vi "WPI_RelayCache.vi"(7 "Operation":T3, 8 "error in (no error)":errorcluster, 9 "RelayDirection":T1, 11 "RelayChannelIn":T2) -> (0 "error out":errorcluster, 2 "Allocated":bool, 3 "RelayChannelOut":T2)   [LabVIEW 2017]
doc: "This software is licensed. Open the labview\\readme\\WPI Robotics Library Open Source License.txt file for more information."
uses:
  <vilib>/Rock Robotics/WPI/Relay/WPI_RelayCacheOp.ctl
  <vilib>/Rock Robotics/SystemInterfaces/DIO/FPGA_DIORelayChannel.ctl
  <vilib>/Rock Robotics/WPI/Relay/WPI_RelayDirection.ctl
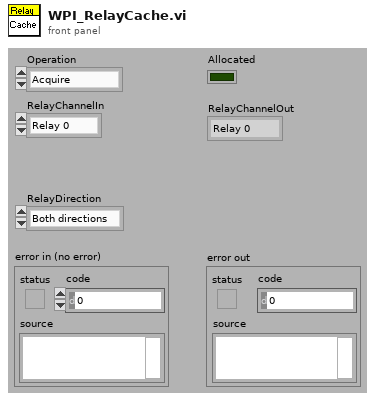
[diagram p1: front panel]
types:
  T1 = typedef "WPI_RelayDirection.ctl" = enum16{"Both directions", "Forward only", "Reverse only"}
  T2 = typedef "FPGA_DIORelayChannel.ctl" = enum8{"Relay 0", "Relay 1", "Relay 2", "Relay 3", "Invalid"}
  T3 = typedef "WPI_RelayCacheOp.ctl" = enum16{"Acquire", "Release", "Status"}
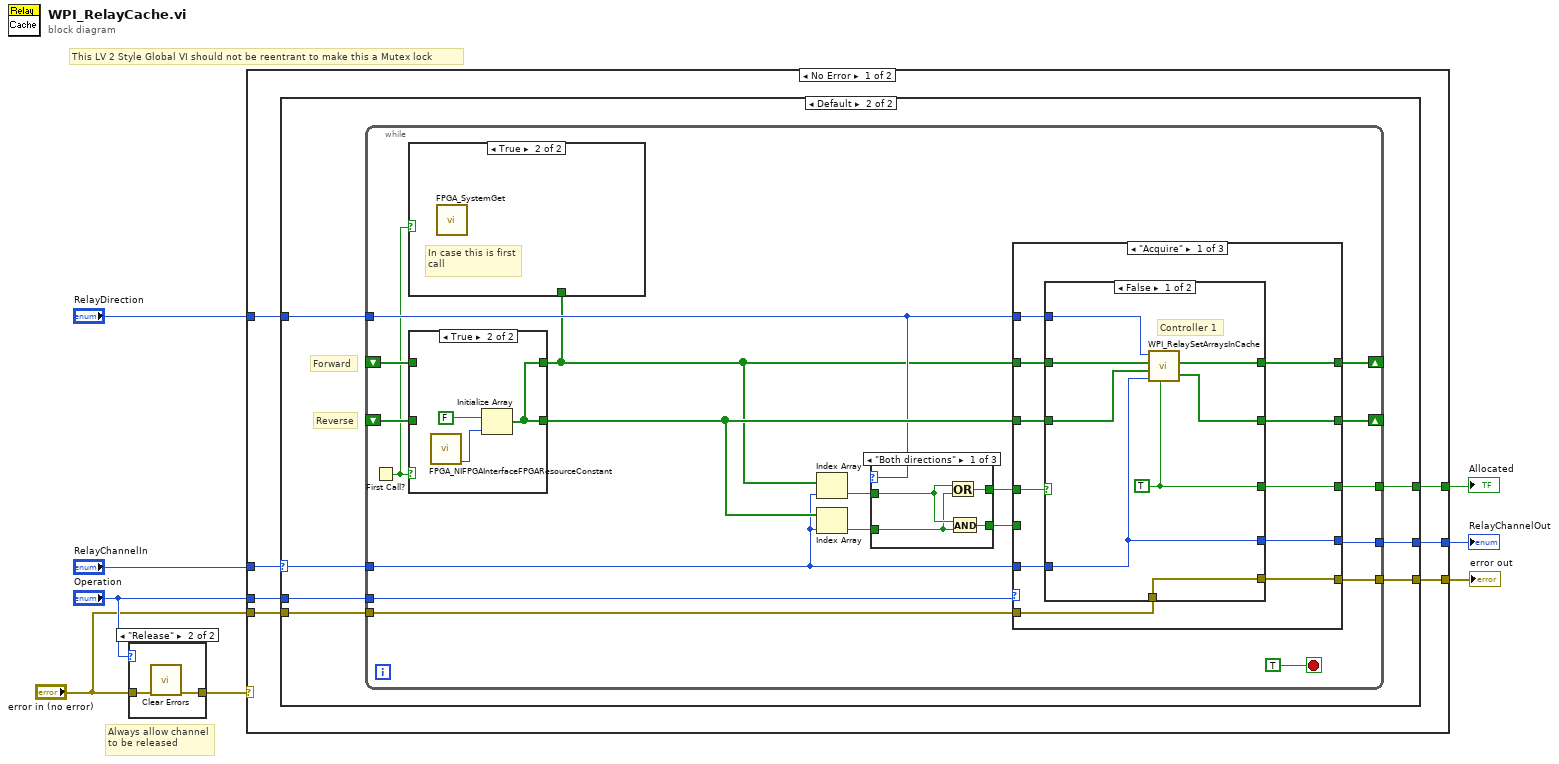
[diagram p0: block diagram]
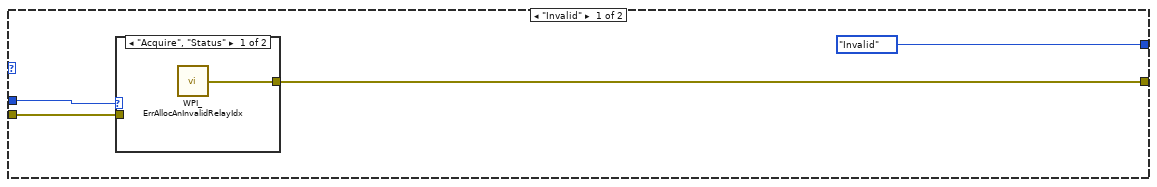
[diagram p2: hidden frame]
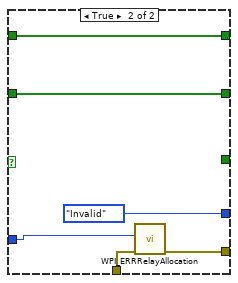
[diagram p6: hidden frame]
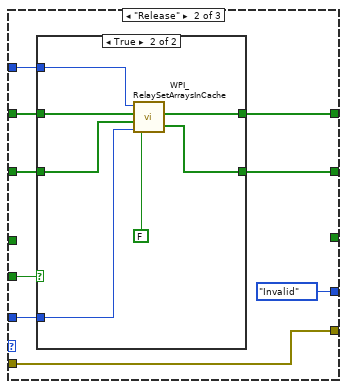
[diagram p7: hidden frame]
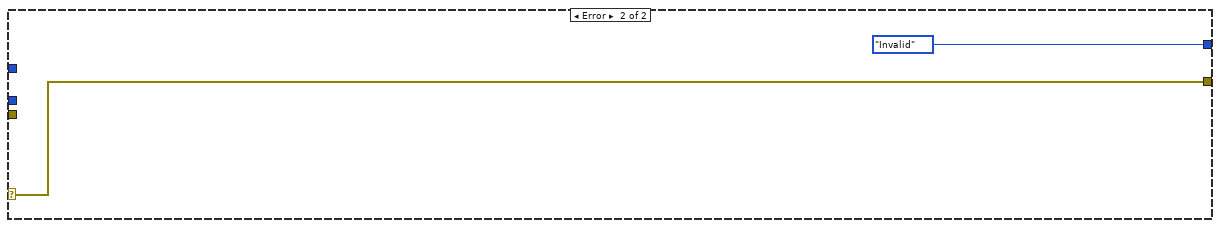
[diagram p12: hidden frame]
diagram:
  # "This LV 2 Style Global VI should not be reentrant to make this a Mutex lock"
  # "Always allow channel to be released"
  n1 = case shown="\"Release\"" "Operation" {
    tunnel: "error in (no error)" -> [w9 w11]
    tunnel: [w9 w10] -> w8
    frame "Acquire", Default {
    }
    frame "Release" {
      n2 = call <vilib>:"Clear Errors.vi"("error in (no error)"=w11) -> ("error out"=w10:errorcluster)  [unwired: 1 in, 5 out]
    }
  }
  n3 = case shown="No Error" w8 {
    selector: w8 -> [_ w110]
    tunnel: "Operation" -> [w18 _]
    tunnel: "RelayChannelIn" -> [w17 _]
    tunnel: [w16 w110] -> w1
    tunnel: [w15 _] -> w5
    tunnel: [w14 FPGA_DIORelayChannel."Invalid" ("RelayChannelOut")] -> w4
    tunnel: "RelayDirection" -> [w13 _]
    tunnel: "error in (no error)" -> [w12 _]
    frame No Error {
      n4 = case shown="Default" w17 {
        selector: w17 -> [_ w26]
        tunnel: w18 -> [w21 w30]
        tunnel: [w20 w29] -> w16
        tunnel: [_ w28] -> w15
        tunnel: [FPGA_DIORelayChannel."Invalid" ("RelayChannelOut") w27] -> w14
        tunnel: w13 -> [_ w25]
        tunnel: w12 -> [w19 w24]
        frame "Invalid" {
          n5 = case shown="\"Acquire\", \"Status\"" w21 {
            tunnel: [w23 _] -> w20
            tunnel: w19 -> [_ _]
            frame "Acquire", "Status" {
              n6 = call <vilib>:"WPI_ErrAllocAnInvalidRelayIdx.vi"() -> ("error out"=w23:errorcluster)
            }
            frame "Release" {
            }
          }
        }
        frame Default {
          # "Forward"
          # "Reverse"
          n7 = while {
            shift-right: [w47] -> _
            shift-left: _ -> [w49]
            tunnel: w30 -> [w48]
            tunnel: w26 -> [w38]
            tunnel: [w46] -> w29
            tunnel: [w45] -> w28
            tunnel: [w42] -> w27
            shift-right: [w40] -> _
            shift-left: _ -> [w41]
            tunnel: w25 -> [w39]
            tunnel: w24 -> [w37]
            stop <- TRUE stop-if-true
            n8 = First Call?() -> (First Call?: T/F=w36:bool)
            n9 = case shown="True" w36 {
              tunnel: w49 -> [w105 _]
              tunnel: [w105 w106] -> w44
              tunnel: w41 -> [w104 _]
              tunnel: [w104 w106] -> w35
              frame False {
              }
              frame True {
                n10 = call <vilib>:"FPGA_NIFPGAInterfaceFPGAResourceConstant.vi"() -> ("NumberOfRelays"=w107:u32)  [unwired: 11 out]
                n11 = Initialize Array(FALSE, w107) -> (w106:bool[])
              }
            }
            n12 = case shown="True" w36 {
              tunnel: w35 -> [_ _]
              frame False {
              }
              frame True {
                # "In case this is first\ncall"
                n13 = call <vilib>:"FPGA_SystemGet.vi"() -> ()  [unwired: 2 in, 10 out]
              }
            }
            n14 = Index Array(array=w35, index=w38) -> (element=w34:bool)
            n15 = Index Array(array=w44, index=w38) -> (element=w33:bool)
            n16 = case shown="\"Both directions\"" w39 {
              tunnel: w34 -> [w52 w54 _]
              tunnel: [w53 w54 w55] -> w32
              tunnel: w33 -> [w51 _ w55]
              tunnel: [w50 w54 w55] -> w31
              frame "Both directions" {
                n17 = Or(x=w52, y=w51) -> (x .or. y?=w50:bool)
                n18 = And(x=w52, y=w51) -> (x .and. y?=w53:bool)
              }
              frame "Forward only" {
              }
              frame "Reverse only" {
              }
            }
            n19 = case shown="\"Acquire\"" w48 {
              tunnel: w44 -> [w62 w89 w103]
              tunnel: [w66 w87 w103] -> w47
              tunnel: w38 -> [w65 w88 w101]
              tunnel: [w64 w81 w99] -> w46
              tunnel: [w63 _ w102] -> w45
              tunnel: w32 -> [_ w86 w102]
              tunnel: [w61 FPGA_DIORelayChannel."Invalid" ("RelayChannelOut") w101] -> w42
              tunnel: [w59 w82 w100] -> w40
              tunnel: w35 -> [w60 w83 w100]
              tunnel: w39 -> [w58 w84 _]
              tunnel: w31 -> [w57 _ _]
              tunnel: w37 -> [w56 w81 w99]
              frame "Acquire" {
                n20 = case shown="False" w57 {
                  tunnel: w62 -> [w73 w80]
                  tunnel: [w72 w80] -> w66
                  tunnel: w65 -> [w71 w75]
                  tunnel: [w67 w76] -> w64
                  tunnel: [w74 _] -> w63
                  tunnel: [w71 FPGA_DIORelayChannel."Invalid" ("RelayChannelOut")] -> w61
                  tunnel: w60 -> [w70 w78]
                  tunnel: [w69 w78] -> w59
                  tunnel: w58 -> [w68 _]
                  tunnel: w56 -> [w67 w77]
                  frame False {
                    w74 = TRUE ("new element/subarray")
                    # "Controller 1"
                    n21 = call <vilib>:"WPI_RelaySetArraysInCache.vi"("Relay Direction"=w68, "forward array  in"=w70, "reverse array in"=w73, "array index"=w71, "new value"=w74) -> ("forward array out"=w69:bool[], "reverse array out"=w72:bool[])
                  }
                  frame True {
                    n22 = call <vilib>:"WPI_ERRRelayAllocation.vi"("error in (no error)"=w77, "RelayChannelIn"=w75) -> ("ERRRelayAllocation"=w76:errorcluster)  [unwired: 9 in]
                  }
                }
              }
              frame "Release" {
                n23 = case shown="True" w86 {
                  tunnel: w89 -> [w91 w96]
                  tunnel: w88 -> [_ w95]
                  tunnel: [w91 w94] -> w87
                  tunnel: w84 -> [_ w98]
                  tunnel: w83 -> [w90 w97]
                  tunnel: [w90 w93] -> w82
                  frame False {
                  }
                  frame True {
                    n24 = call <vilib>:"WPI_RelaySetArraysInCache.vi"("Relay Direction"=w98, "forward array  in"=w97, "reverse array in"=w96, "array index"=w95, "new value"=FALSE ("new element/subarray")) -> ("forward array out"=w93:bool[], "reverse array out"=w94:bool[])
                  }
                }
              }
              frame "Status" {
              }
            }
          }
        }
      }
    }
    frame Error {
    }
  }
  "Allocated" <- w5
  "error out" <- w1
  "RelayChannelOut" <- w4
